vi "meter_to_feet.vi"(1 "Meter":dbl format="%#.3f") -> (0 "Feet":dbl format="%#.3f")   [LabVIEW 2013]
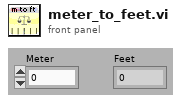
[diagram p1: front panel]
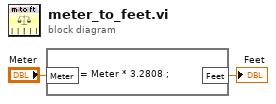
[diagram p0: block diagram]
diagram:
  n1 = formula code="Feet = Meter * 3.2808 ;"("Meter"="Meter") -> ("Feet"=→"Feet":dbl)
